vi "logging loop.vi"(8 "error in":errorcluster, 9 "Maker":T1(ring), 10 "Saving":refnum<vi>, 11 "Log queue":refnum<queue>) -> (0 "error out":errorcluster)   [LabVIEW 2016]
uses:
  Queue Message Handler/Message Cluster.ctl
  Control/Settings.ctl
  Control/port config.ctl
  <vilib>/LabVIEW Interface for Arduino/Type Defs/Board Type.ctl
  <vilib>/Utility/file.llb/Write Delimited Spreadsheet (string).vi
  Queue Message Handler/Message Queue.lvlib
  <vilib>/LabVIEW Interface for Arduino/LabVIEW Interface for Arduino.lvlib
panel:
  out "Result file":string
  in  "File name":string="test"
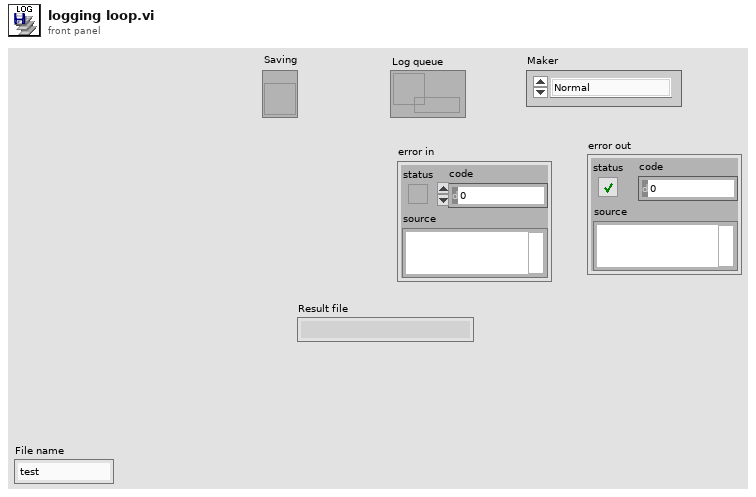
[diagram p1: front panel]
types:
  T1 = enum16{"Normal", "Blink", "Double blink", "Mozart ", "High focus", "favourite music", "Smile"}
  T2 = typedef "Settings.ctl" = cluster{"Port":T3, "Sample Rate (HZ)":u16, "Samples to Read":u16, "Input Pin":u8, "File path saved":path}
  T3 = typedef "port config.ctl" = cluster{"Port Name":refnum<visa-resource-name>, "Board Type":T4, "Baud Rate":u32}
  T4 = typedef "LabVIEW Interface for Arduino.lvlib/Board Type.ctl" = enum16{"Uno", "Dimuelanove w/Atmega 328", "Mega 2560"}
  T5 = enum16{"open", "replace", "create", "open or create", "replace or create", "replace or create with confirmation"}
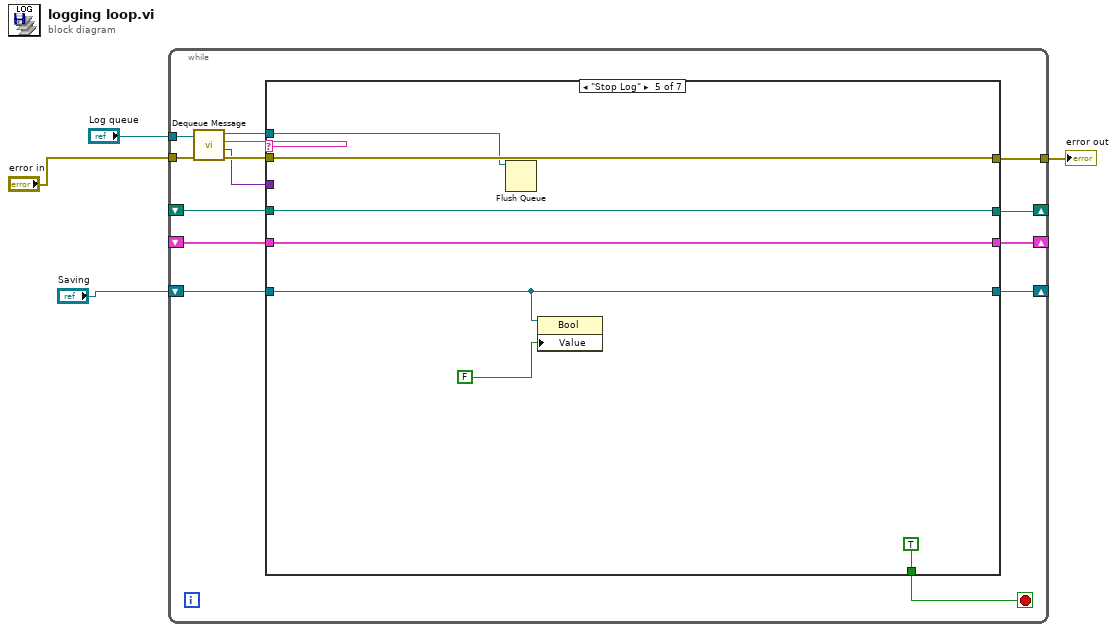
[diagram p0: block diagram]
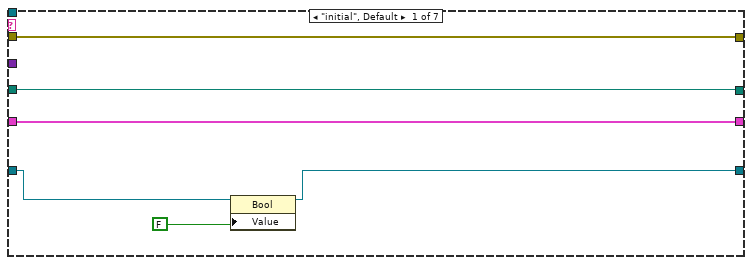
[diagram p2: hidden frame]
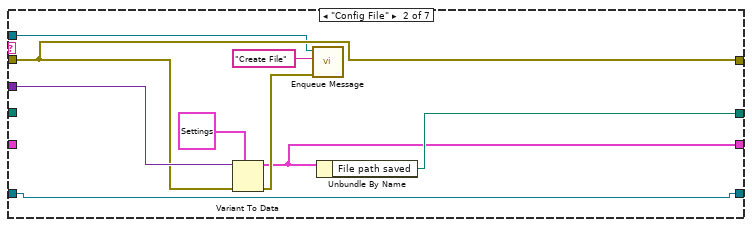
[diagram p3: hidden frame]
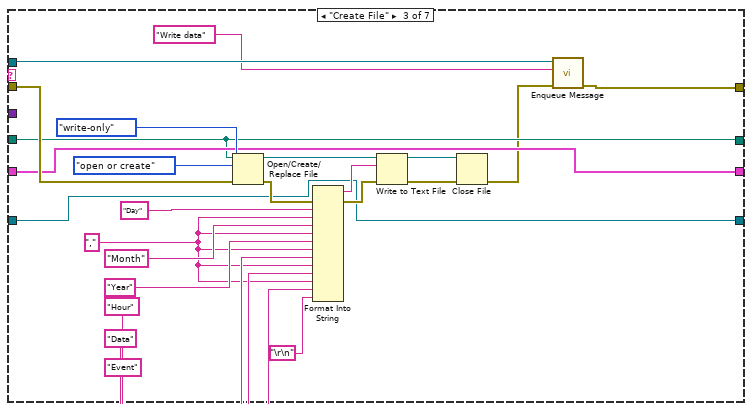
[diagram p4: hidden frame]
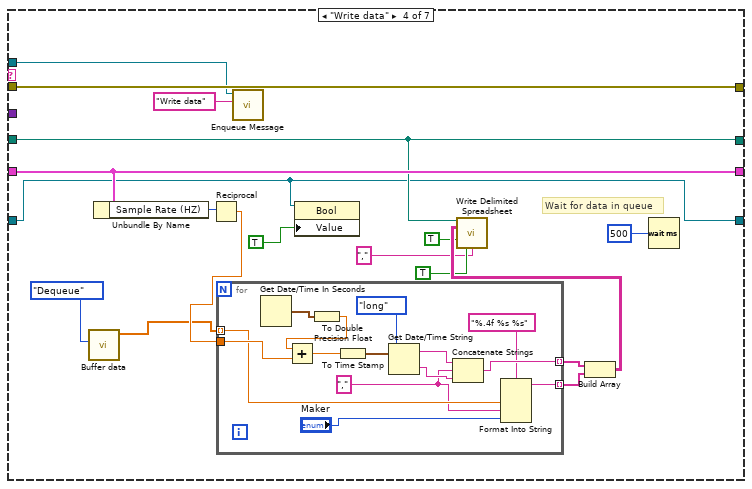
[diagram p5: hidden frame]
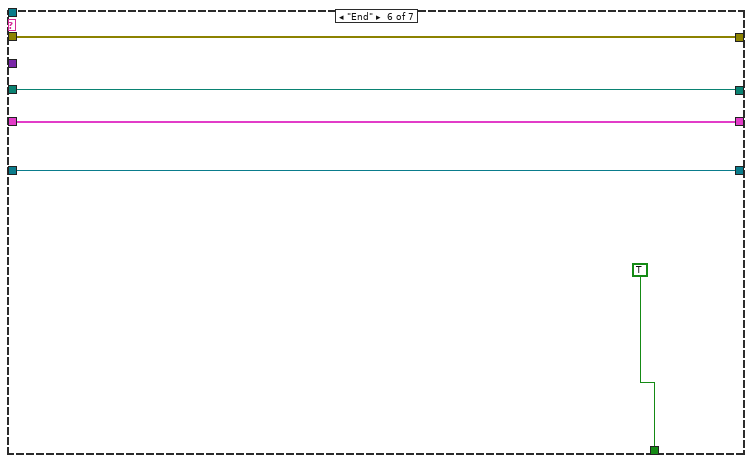
[diagram p6: hidden frame]
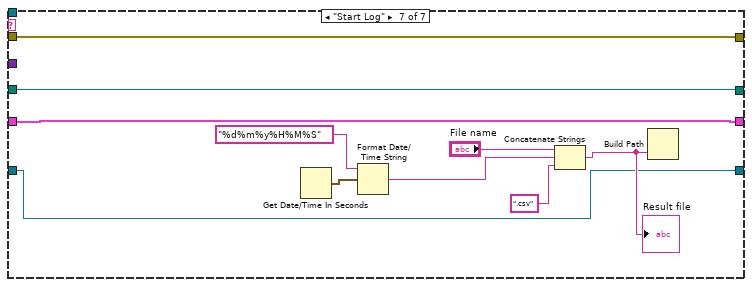
[diagram p7: hidden frame]
diagram:
  n1 = while {
    tunnel: "Log queue" -> [w17]
    tunnel: "error in" -> [w16]
    shift-right: [w13] -> _
    shift-left: _ -> [w12]
    tunnel: [w9] -> w2
    shift-right: [w8] -> _
    shift-left: _ -> [w7]
    shift-right: [w5] -> _
    shift-left: "Saving" -> [w6]
    stop <- w10 stop-if-true
    n2 = call "Dequeue Message.vi"("error in (no error)"=w16, "Message Queue"=w17) -> ("error out"=w15:errorcluster, "Message Data"=w14:variant, "Message"=w18:string, "dup Message Queue"=w11:refnum<queue>)  [unwired: 6 in]
    n3 = case shown="\"Stop Log\"" w18 {
      tunnel: w15 -> [w23 w31 w44 w75 w95 w99 w104]
      tunnel: w14 -> [_ w32 _ _ _ _ _]
      tunnel: [w24 w27 w38 w67 w96 w101 w105] -> w13
      tunnel: w12 -> [w24 _ w38 w67 w96 w101 w105]
      tunnel: w11 -> [_ w29 w46 w62 w93 _ _]
      tunnel: [_ _ _ _ TRUE TRUE _] -> w10
      tunnel: [w23 w31 w41 w75 w95 w99 w104] -> w9
      tunnel: [w22 w26 w40 w74 w94 w98 w103] -> w8
      tunnel: w7 -> [w22 _ w40 w74 w94 w98 w103]
      tunnel: w6 -> [w20 w25 w34 w59 w91 w97 w102]
      tunnel: [w19 w25 w34 w59 w91 w97 w102] -> w5
      frame "initial", Default {
        n4 = property class="Bool"(reference=w20, "Value"=FALSE) -> (reference out=w19:refnum<vi>)  [unwired: 1 in, 1 out]
      }
      frame "Config File" {
        n5 = Variant To Data(error in=w31, type=T2 {"Port"={"Port Name"="", "Board Type"=enum."Uno", "Baud Rate"=115200}, "Sample Rate (HZ)"=100, "Samples to Read"=50, "Input Pin"=0, "File path saved"=path ""} ("Settings out"), Variant=w32) -> (data=w26:T2, error out=w30:errorcluster)
        n6 = call "Enqueue Message.vi"("error in (no error)"=w30, "Message"="Create File", "Message Queue"=w29) -> ()  [unwired: 7 in, 2 out]
        n7 = Unbundle By Name(w26) -> ("File path saved"=w27:path)
      }
      frame "Create File" {
        w49 = ","
        n8 = Open/Create/Replace File(file path (use dialog)=w38, error in=w44, operation (0:open)=T5."open or create", access (0:read/write)=enum16{"read/write", "read-only", "write-only"}."write-only") -> (refnum out=w35:refnum<file>, error out=w43:errorcluster)  [unwired: 2 in, 1 out]
        n9 = Format Into String(error in=w43, "Day", w49, "Month", w49, "Year", w49, "Hour", w49, "Data", w49, "Event", "\r\n") -> (resulting string=w55:string, error out=w42:errorcluster)  [unwired: 2 in]
        n10 = Write to Text File(file (use dialog)=w35, text=w55, error in=w42) -> (refnum out=w37:refnum<file>, error out=w39:errorcluster)  [unwired: 1 in, 1 out]
        n11 = Close File(refnum=w37, error in=w39) -> (error out=w36:errorcluster)  [unwired: 1 out]
        n12 = call "Enqueue Message.vi"("error in (no error)"=w36, "Message"="Write data", "Message Queue"=w46) -> ("error out"=w41:errorcluster)  [unwired: 7 in, 1 out]
      }
      frame "Write data" {
        # "Wait for data in queue"
        n13 = call "Buffer data.vi"("Command"=enum16{"Create", "Enqueue", "Dequeue", "Clear"}."Dequeue") -> ("Data out"=w70:dbl[])  [unwired: 9 in, 1 out]
        n14 = Unbundle By Name(w74) -> ("Sample Rate (HZ)"=w73:u16)
        n15 = Reciprocal(x=w73) -> (1/x=w72:dbl)
        n16 = for {
          tunnel: w70 -> [w86] mode=indexing
          tunnel: w72 -> [w87]
          tunnel: [w81] -> w68 mode=indexing
          tunnel: [w80] -> w69 mode=indexing
          w79 = ","
          n17 = Get Date/Time In Seconds() -> (seconds since 1Jan1904=w89:timestamp)
          n18 = To Double Precision Float(number=w89) -> (double precision float=w88:dbl)
          n19 = Add(x=w88, y=w87) -> (x+y=w85:dbl)
          n20 = To Time Stamp(1:w85) -> (0:w84:timestamp)
          n21 = Get Date/Time String(date format (0)=enum16{"short", "long", "abbreviated"}."long", seconds (now)=w84) -> (date string=w83:string, time string=w82:string)  [unwired: 1 in]
          n22 = Concatenate Strings(w83, w79, w82) -> (w80:string)
          n23 = Format Into String(format string="%.4f %s %s", w86, w79, "Maker") -> (resulting string=w81:string)  [unwired: 2 in, 1 out]
        }
        n24 = call "Enqueue Message.vi"("Message"="Write data", "Message Queue"=w62) -> ()  [unwired: 8 in, 2 out]
        n25 = property class="Bool"(reference=w59, "Value"=TRUE) -> ()  [unwired: 1 in, 2 out]
        n26 = Build Array(w69, w68) -> (w66:string[][])
        n27 = call-poly <vilib>:"Write Delimited Spreadsheet.vi"("file path (dialog if empty)"=w67, "2D data"=w66, "append to file? (new file:F)"=TRUE, "transpose? (no:F)"=TRUE, "delimiter (\\t)"="," ("delimiter (\\t)")) -> ()  [unwired: 9 in, 2 out]
        n28 = Wait (ms)(milliseconds to wait=u32 500) -> ()  [unwired: 1 out]
      }
      frame "Stop Log" {
        n29 = Flush Queue(queue=w93) -> ()  [unwired: 1 in, 3 out]
        n30 = property class="Bool"(reference=w91, "Value"=FALSE) -> ()  [unwired: 1 in, 2 out]
      }
      frame "End" {
      }
      frame "Start Log" {
        n31 = Get Date/Time In Seconds() -> (seconds since 1Jan1904=w107:timestamp)
        n32 = Format Date/Time String(time format string (%c)="%d%m%y%H%M%S", seconds (now)=w107) -> (date/time string=w106:string)  [unwired: 1 in]
        n33 = Concatenate Strings("File name", w106, ".csv") -> (w108:string)
        "Result file" <- w108
        n34 = Build Path(name or relative path=w108) -> ()  [unwired: 1 in, 1 out]
      }
    }
  }
  "error out" <- w2
